vi "BeamAnalyzer.vi"() -> ()   [LabVIEW 2021]
uses:
  <vilib>/vision/Image Controls.llb/IMAQ Image.ctl
  <vilib>/userdefined/High Color/IMAQdx.ctl
  <vilib>/vision/driver/NI_Vision_Acquisition_Software.lvlib
  <vilib>/Utility/TDMS File Viewer/NI_TDMS File Viewer.lvlib
panel:
  in  "tabControl":T1(tab)
  in  "resetOrigin":bool
  in  "setOrigin":bool
  out "lastBufferNumber":u32
  out "imageRows":i32 caption="Rows"
  out "imageCols":i32 caption="Columns"
  out "Trials":i32
  in  "verticalTermPars":cluster{"max iteration":dbl, "tolerance":dbl}={"max iteration"=20.0, "tolerance"=0.0001} caption="Termination \nParameters"
  out "exposureTimeStatus":bool caption="Status"
  in  "aboutButton":bool
  out "vetFitLED":bool
  out "horzFitLED":bool
  in  "maxTrialNumber":i32=10 caption="Max Trial Number"
  out "followCyLED":bool
  out "followCxLED":bool
  in  "exposureTime":dbl caption="Exposure Time" format="%#_6ps"
  out "minMax":u16[](array[numeric]) caption="Min Max Intensities"
  in  "intesityRangeTreshold":dbl=0.33 caption="Intesity Range\nTreshold Fraction"
  in  "fitCol":i32=640
  in  "followCy":bool
  in  "followCx":bool
  in  "stop":bool
  in  "blahButton":bool
  in  "percentageMaxIntensity":dbl=75.0 caption="Percentage Max Intensity" format="%#_g%%"
  out "imageViewer":T2(plugin-control)
  in  "setExposureButton":bool
  in  "horizontalFitButton":bool
  out "horizontal FitPlot":cluster{"xAxis":dbl[], "horizontalFitY":dbl[]}[](graph)
  in  "horizontalTermPars":cluster{"max iteration":dbl, "tolerance":dbl}={"max iteration"=20.0, "tolerance"=0.0001} caption="Termination \nParameters"
  out "horizontalBestFitPars":dbl[](array[numeric]) caption="Best Fit Pars" format="%#_6p"
  out "horizontalFitCovariance":dbl[][](array[numeric]) caption="Covariance" format="%#_6p"
  out "verticalFitPlot":T3(graph)
  out "verticalBestFitPars":dbl[](array[numeric]) caption="Best Fit Pars" format="%#_6p"
  in  "verticalFitButton":bool
  in  "fitRow":i32=480
  out "verticalFitError":errorcluster
  out "horizontalFitError":errorcluster
  in  "saveCurrentImage":bool
  in  "baseName":string="blah"
  in  "basePath":path=path "./"
  out "last Image filename":string
  out "verticalFitCovariance":dbl[][](array[numeric]) caption="Covariance" format="%#_6p"
  out "Cx":dbl caption="X" format="%#_6pm"
  out "Cy":dbl caption="Y" format="%#_6pm"
  out "Y":dbl format="%#_4pm"
  out "X":dbl format="%#_4pm"
  out "centroidCoords":cluster{"Cx":dbl, "Cy":dbl} caption="Centroid Coords" {"Cy" format="%u px"; "Cx" format="%u px"}
  out "wx":dbl format="%#_4pm"
  out "wy":dbl format="%#_4pm"
  out "lumberingLED":bool
  in  "runChartButton":bool
  out "last log filename":string
  in  "log basePath":path
  in  "logBaseName":string="blah"
  in  "logDataButton":bool
  out "wx_wyPlot":cluster{"Numeric":dbl, "Numeric":dbl}(graph)={"Numeric"=24.443322449703377, "Numeric"=50.238781903198756}
  out "CyPlot":dbl(graph)=-0.6586166381835937
  out "CxPlot":dbl(graph)=-1.7079547119140623
  in  "AlliedVisionImageGrabPatch":bool=TRUE
  out "cameraSession":T4 caption="Session Out"
  out "imageBuffer":T2
  in  "reticleColor":u32(colorbox)=3800611 caption="Reticle Pattern Color"
  in  "units":enum32{"um", "mm", "cm"}(radio)
  in  "maxExposureTime":dbl=0.1 caption="Max Exp. Time" format="%#_4ps"
  in  "minExposureTime":dbl=6e-06 caption="Min Exp. Time" format="%#_4ps"
  out "intensityRangeMax":u16
  out "errorExposureTime":errorcluster
  out "errorCameraConfig":errorcluster
  out "errorImageGrab":errorcluster
  out "plotUnitsPrefix":dbl=1000.0
  in  "exposuretimeUnitsPrefix":dbl=1000000.0 caption="Exp.  Time Units Prefix" format="%#_6p"
  out "vendorNameModelName":string
  out "errorCameraParsRequest":errorcluster
  out "IPAddress":string
  in  "nbits":u16=14 min=4 max=15
  in  "pixelSize":dbl=3e-05 caption="Calibrated Pixel Size" format="%#_6pm"
  in  "device":string(combo)="cam1"
  out "xAxis":dbl[](array[numeric])
  out "yAxis":dbl[](array[numeric])
  out "colsOffset":i32
  out "rowsOffset":i32
  out "rowArray":u16[](array[numeric])
  out "colArray":u16[](array[numeric])
  out "verticalFitY":dbl[](array[numeric])
  out "horizontalFitY":dbl[](array[numeric])
  out "centroidError":errorcluster
  out "imageDecorated":T2
  out "TDMS_Location":path
  out "TDMS_Handle":refnum<k34>
  out "errorTDMS_LogClose":errorcluster
  out "errorTDMS_LogOpen":errorcluster
  out "yAxisScaled":dbl[](array[numeric])
  out "xAxisScaled":dbl[](array[numeric])
  out "errorTDMS_LogWrite":errorcluster
  # "I0"
  # "AU/px"
  # "m"
  # "x0"
  # "m"
  # "w0"
  # "AU/px"
  # "I1"
  # "Exposure Setting"
  # "Centroid"
  # "Image Statistics"
  # "Save Current Livefeed Image"
  # "AU/px"
  # "I0"
  # "m"
  # "x0"
  # "w0"
  # "m"
  # "AU/px"
  # "I1"
  # "Spot Radii"
  # "Centroid Coords"
  # "Camera Configuration"
  # "Model"
  # "Plot Configuration"
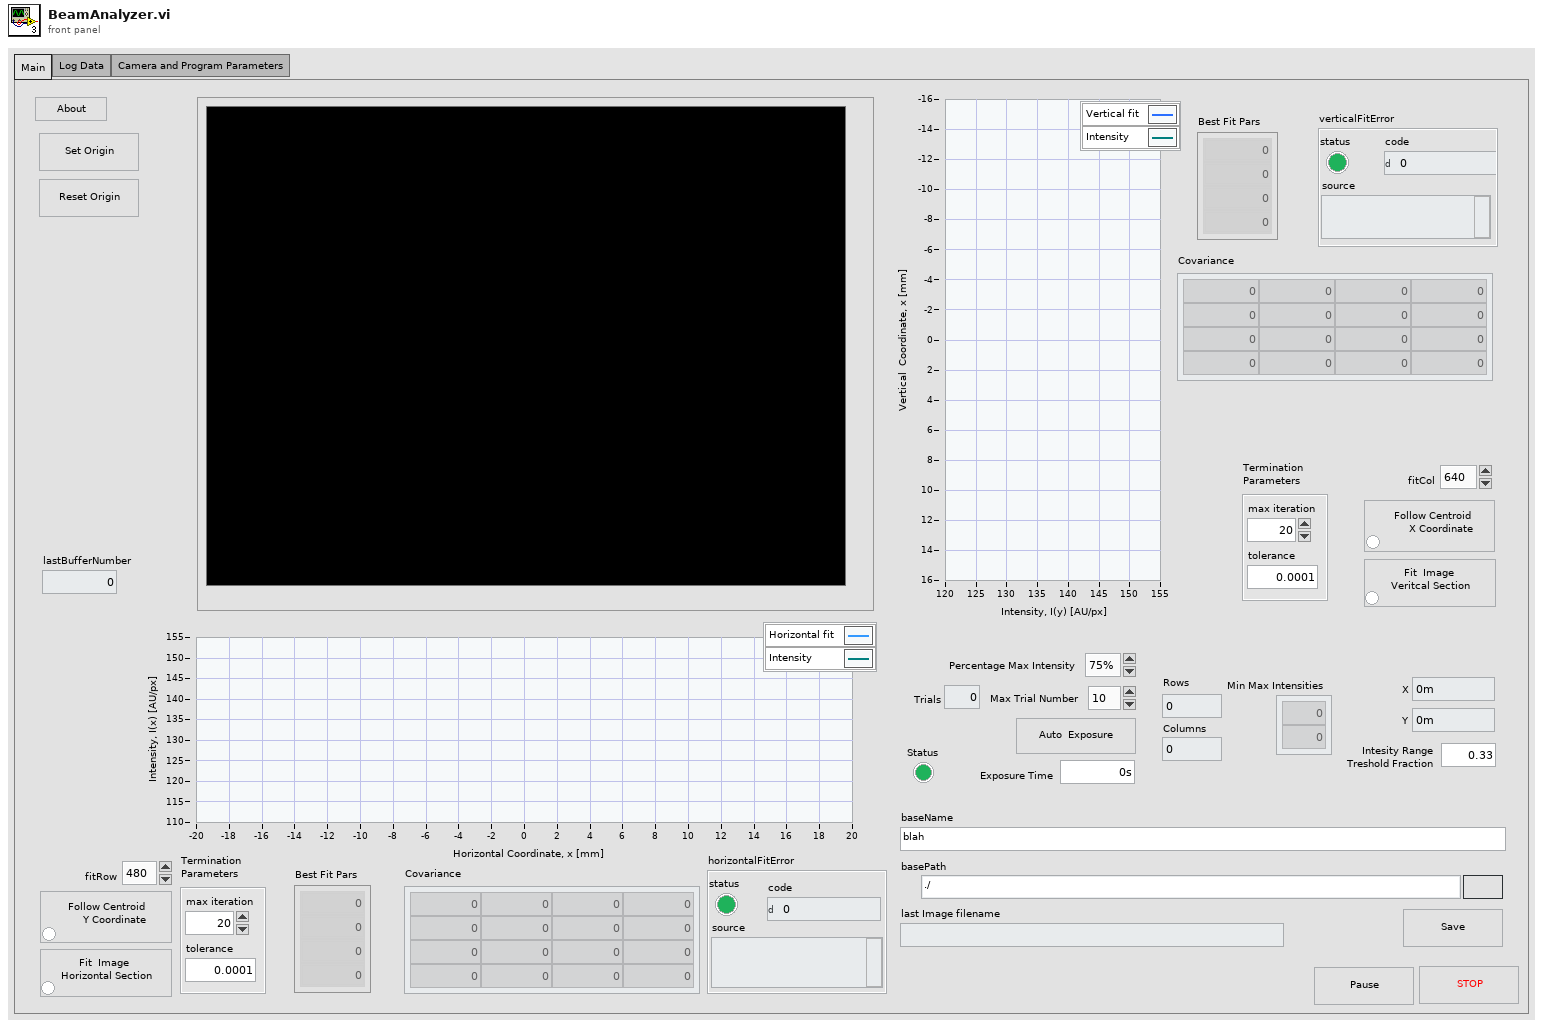
[diagram p1: front panel]
types:
  T1 = enum32{"Main", "Log Data", "Camera and Program Parameters"}
  T2 = typedef "IMAQ Image.ctl" = refnum<image>
  T3 = cluster{"best nonlinear fit":dbl[], "yAxis":dbl[]}[]
  T4 = typedef "IMAQdx.ctl" = refnum<k21>
  T5 = enum32{"Fit", "Log Data", "Camera and Program Parameters"}
  T6 = enum32{"Fit", "Log Data", "Hardware  Parameters"}
  T7 = enum16{"open", "open or create", "create or replace", "create", "open (read-only)"}
  T8 = cluster{"xAxisScaled":dbl[], "horizontalFitY":dbl[]}
  T9 = cluster{"xAxisScaled":dbl[], "horizontalFitY":dbl[]}[]
  T10 = cluster{"verticalFitY":dbl[], "yAxisScaled":dbl[]}
  T11 = cluster{"verticalFitY":dbl[], "yAxisScaled":dbl[]}[]
  T12 = typedef "NI_Matrix.lvlib/RealMatrix.ctl" = dbl[][]
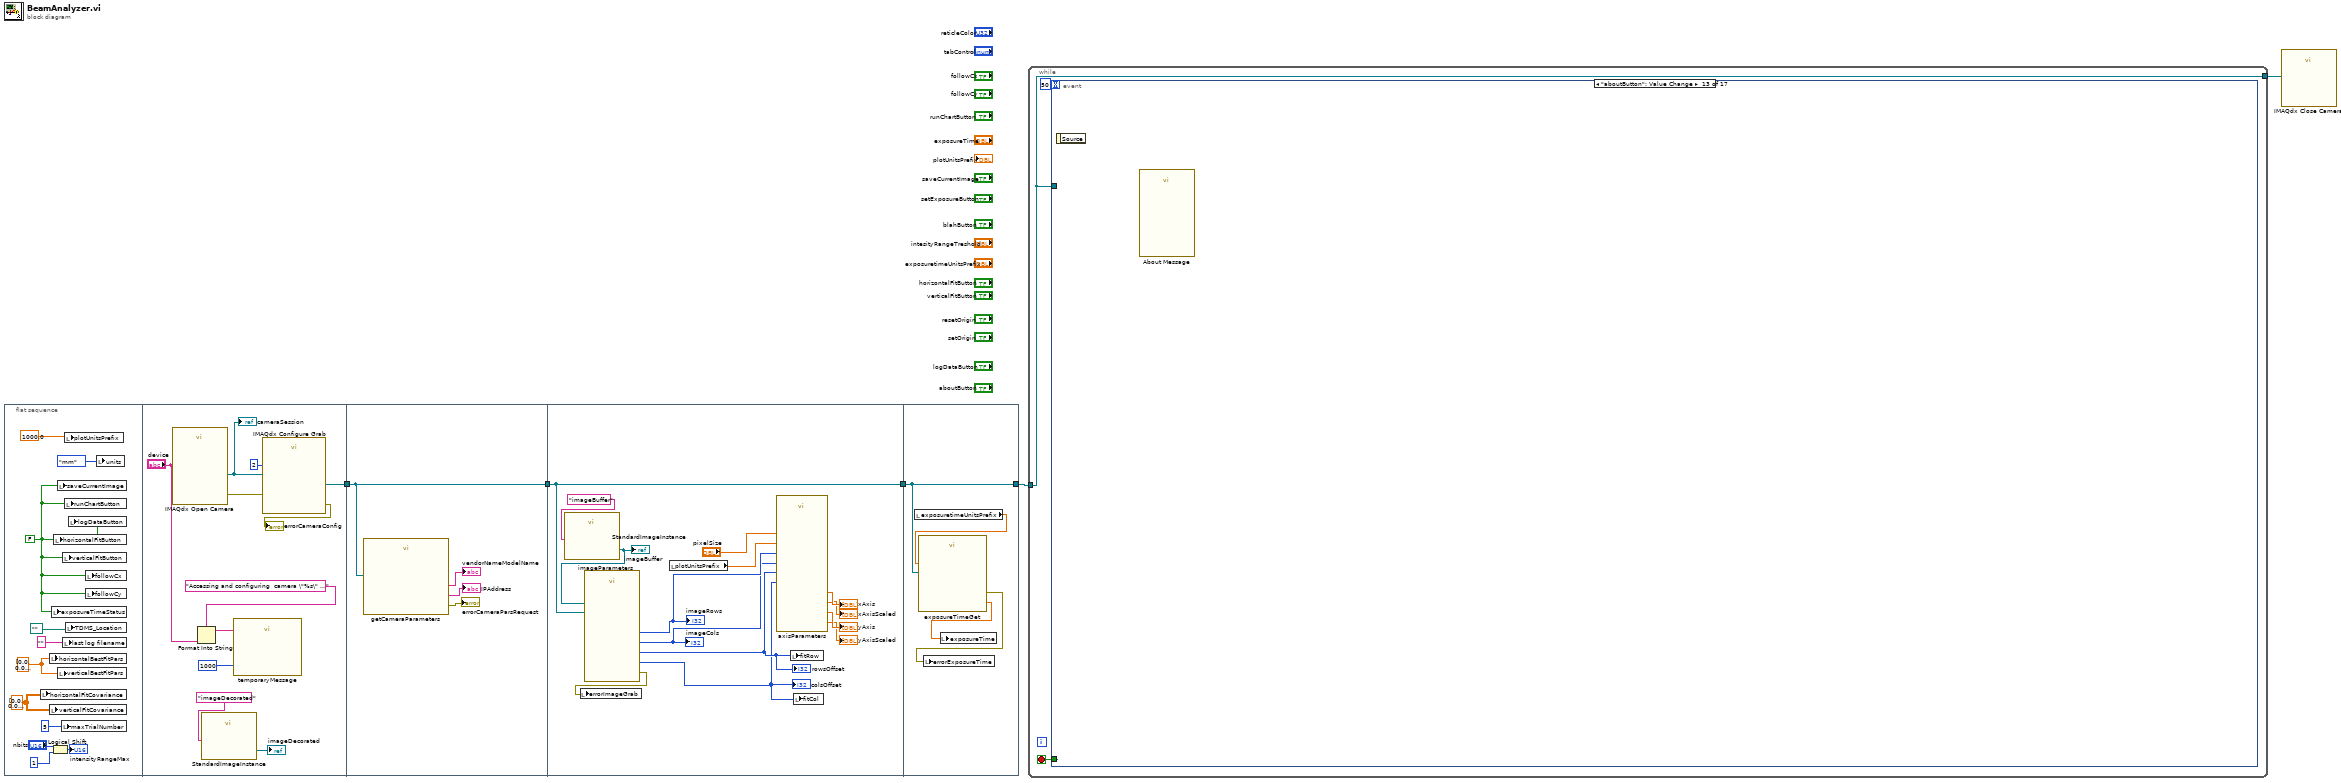
[diagram p0: block diagram]
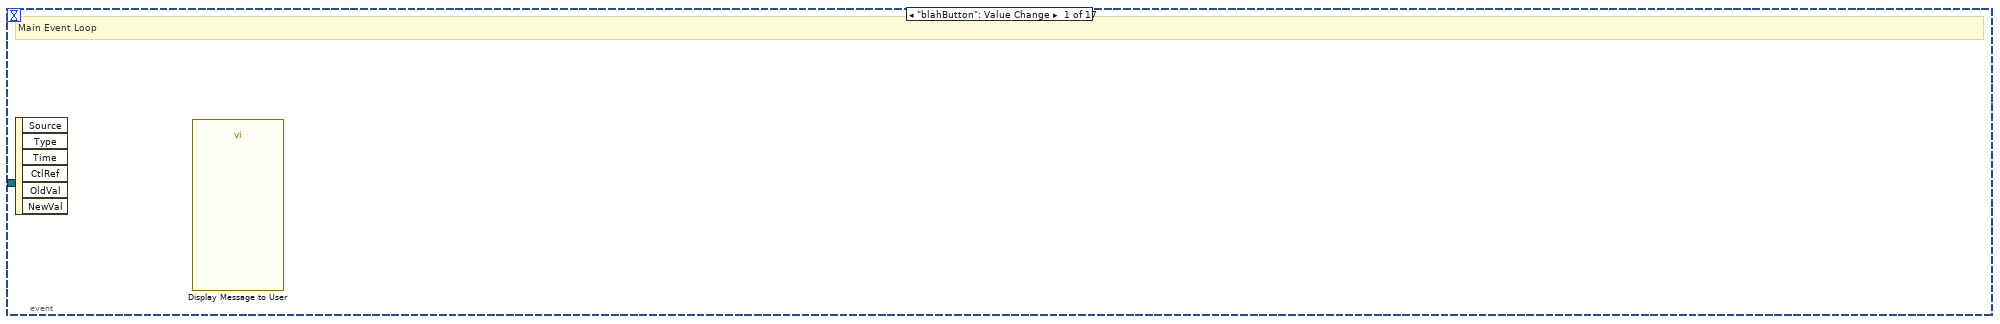
[diagram p2: hidden frame]
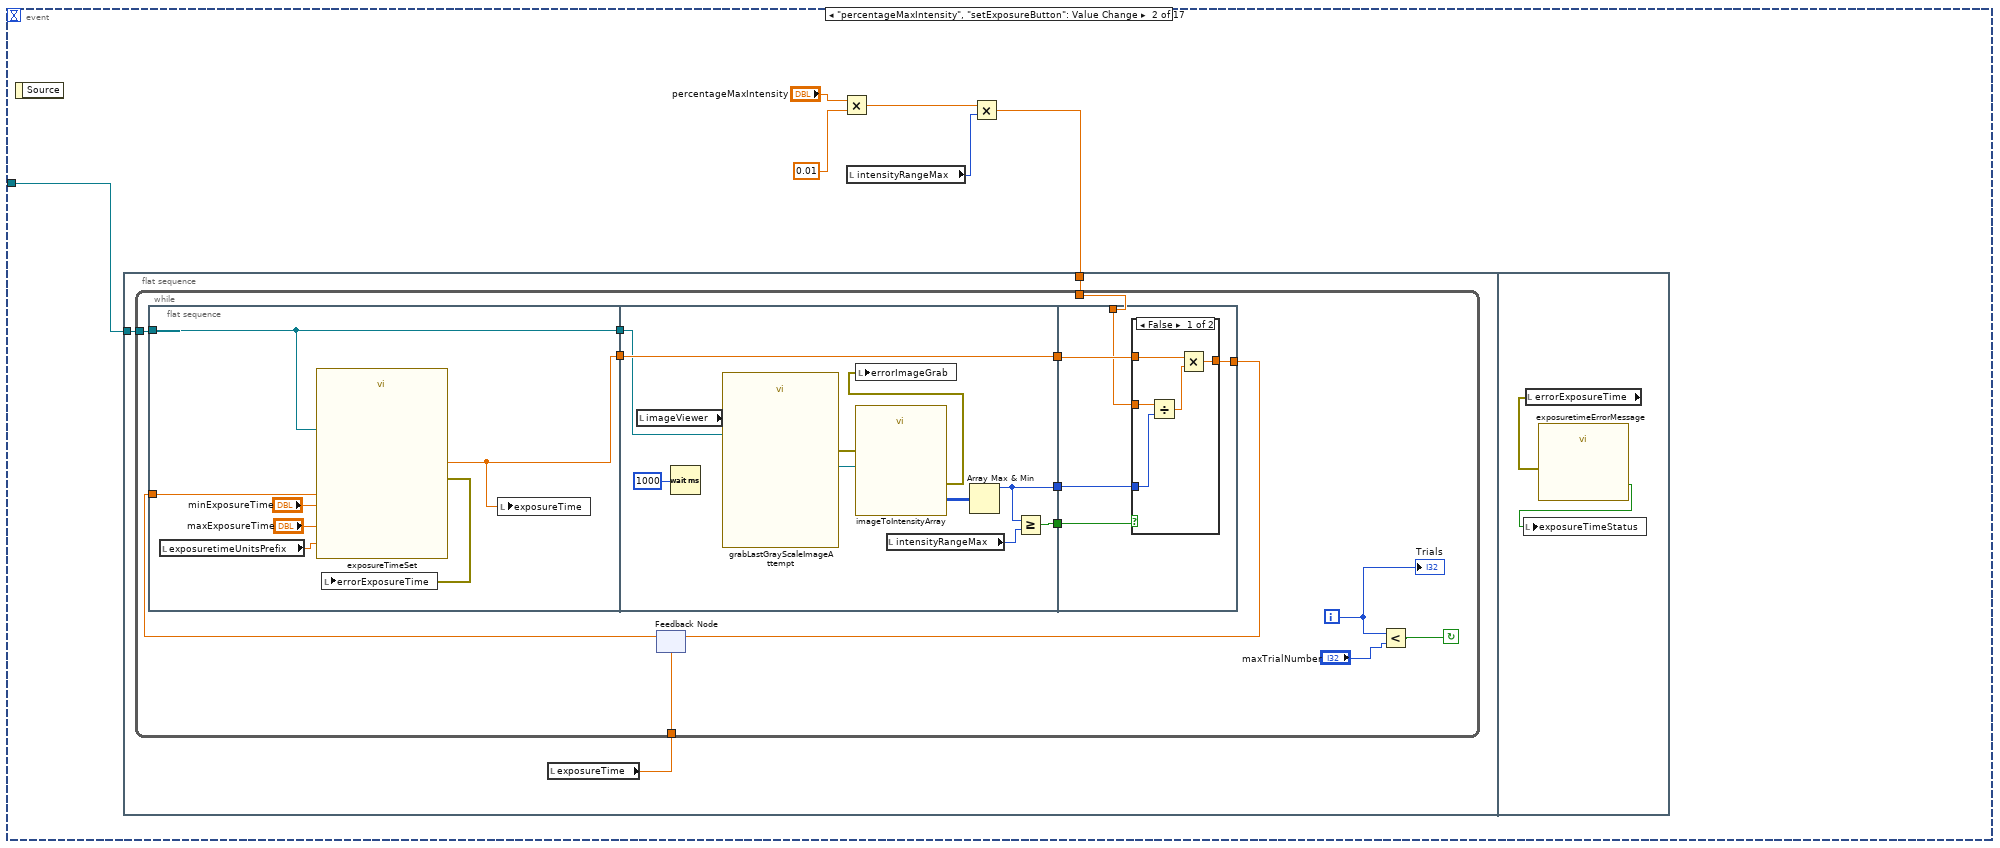
[diagram p3: hidden frame]
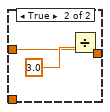
[diagram p4: hidden frame]
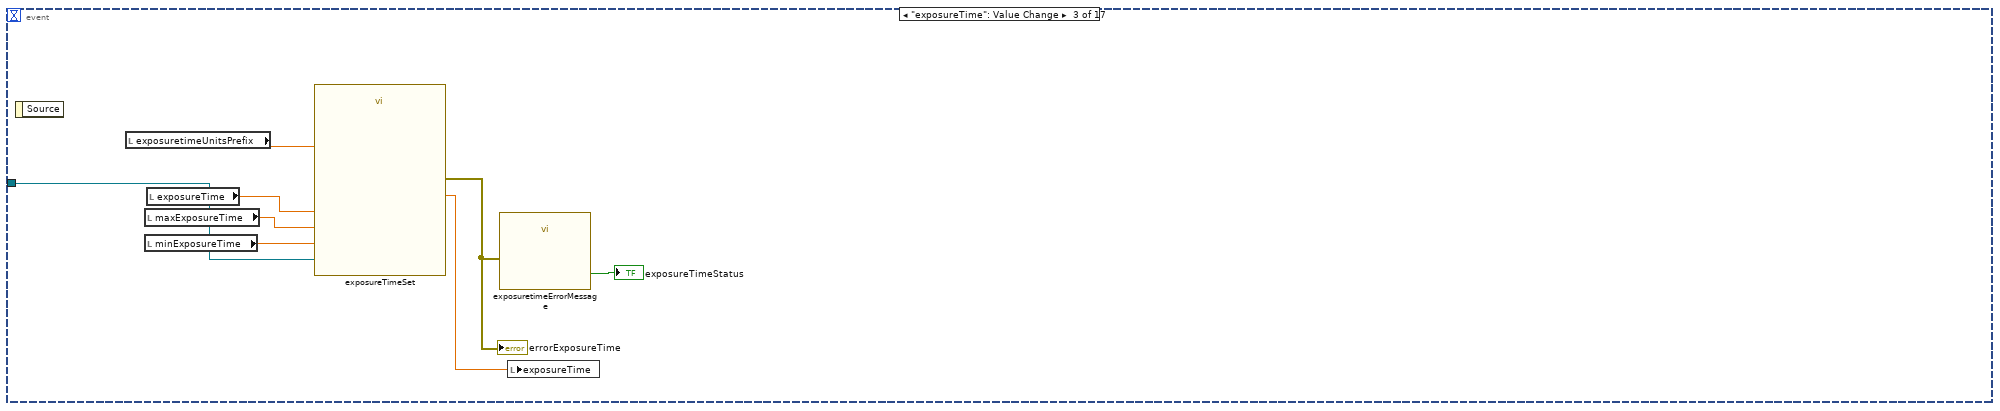
[diagram p5: hidden frame]
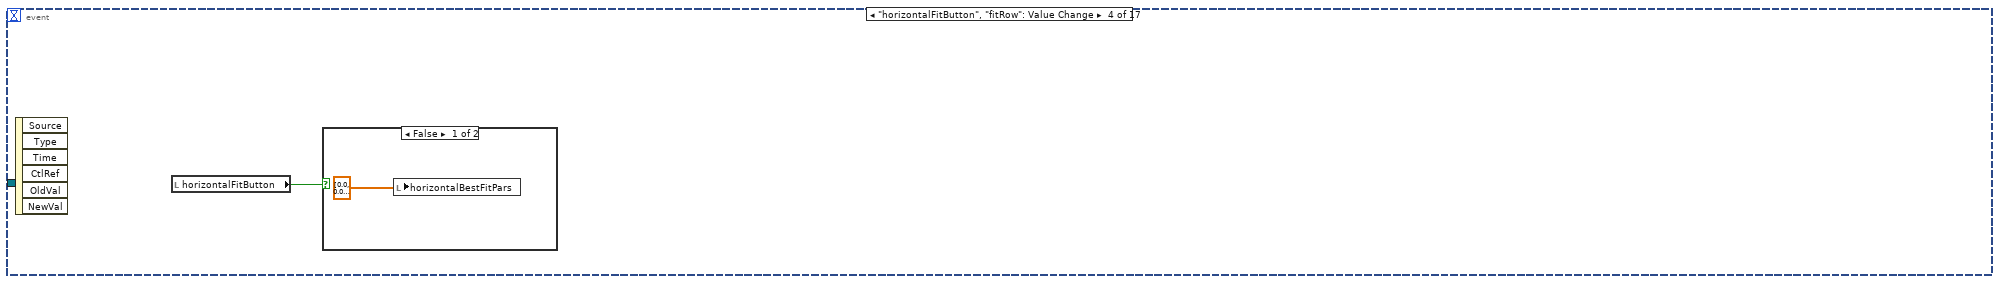
[diagram p6: hidden frame]
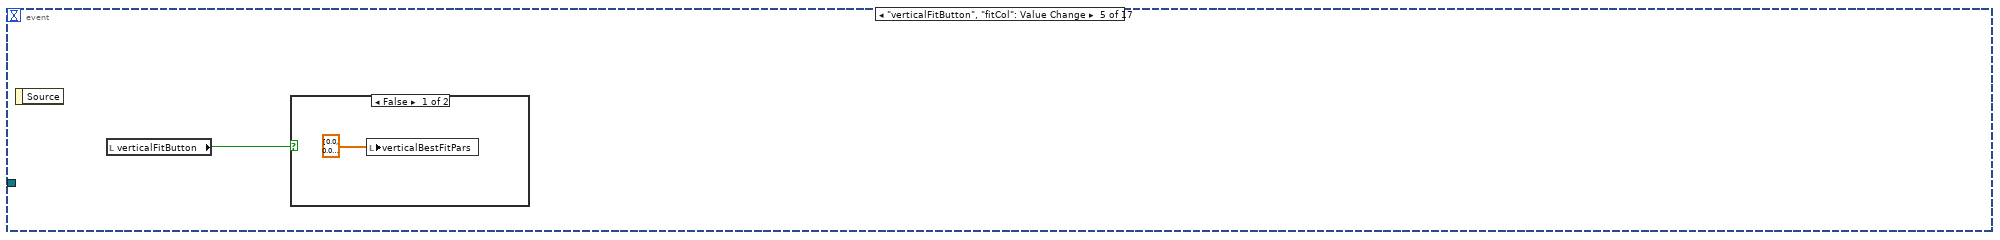
[diagram p8: hidden frame]
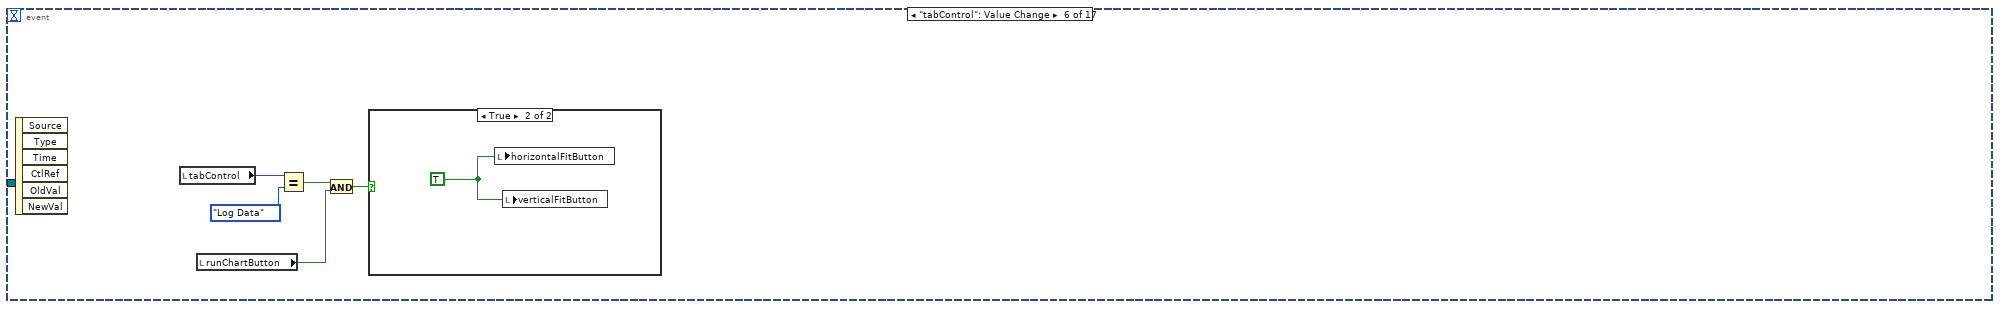
[diagram p10: hidden frame]
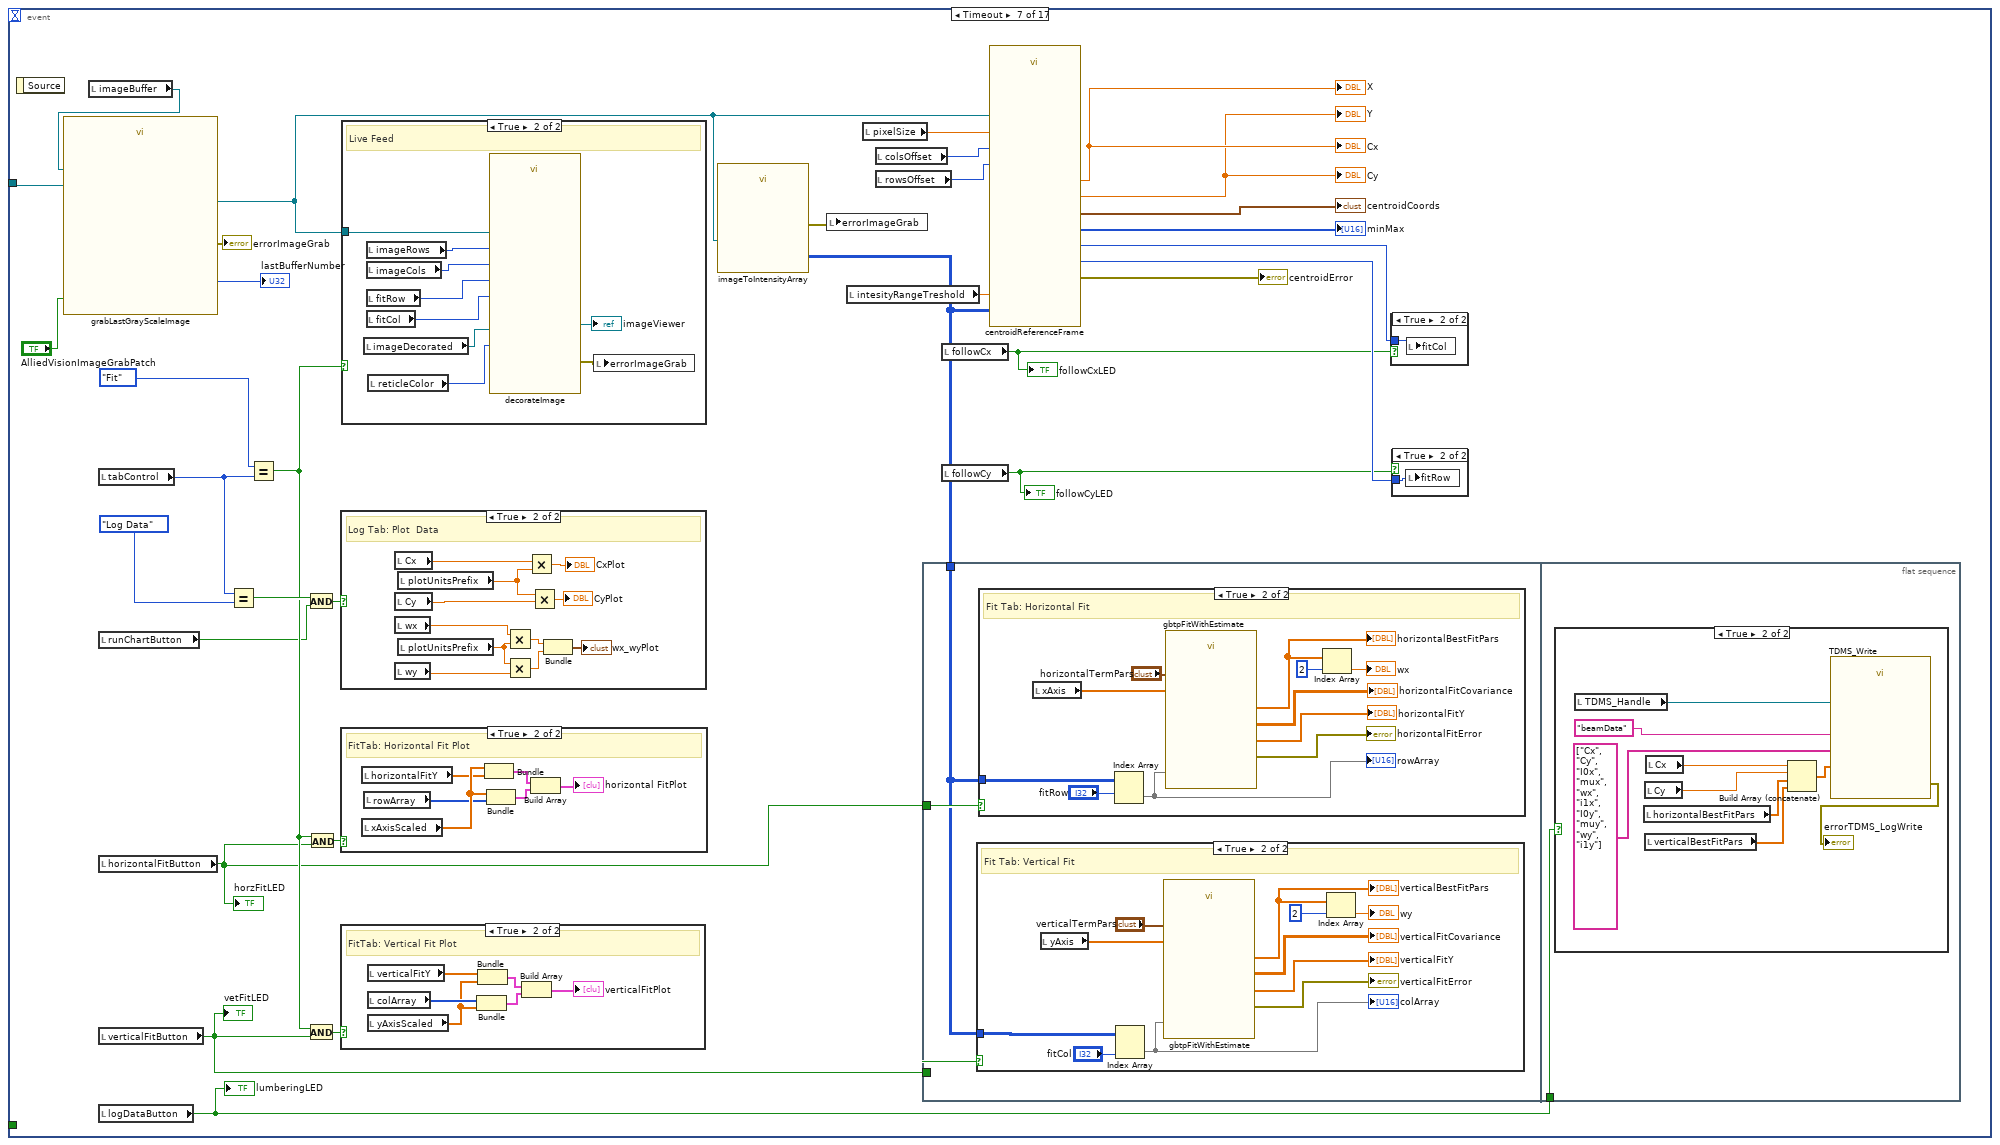
[diagram p12: hidden frame]
diagram:
  n1 = flat-sequence {
    tunnel: [w23] -> w3
    tunnel: [w28] -> w4
    tunnel: w3 -> [w28]
    tunnel: [w42] -> w5
    tunnel: w4 -> [w42]
    tunnel: [w46] -> w2
    tunnel: w5 -> [w46]
    frame #0 {
      w13 = dbl[][] [[0.0, 0.0, 0.0, 0.0], [0.0, 0.0, 0.0, 0.0], [0.0, 0.0, 0.0, 0.0], [0.0, 0.0, 0.0, 0.0]] ("horizontalFitCovariance")
      w14 = dbl[] [0.0, 0.0, 0.0, 0.0, 0.0] ("horizontalBestFitPars")
      w11 = FALSE
      n2 = local write "horizontalFitCovariance"(w13) -> ()
      n3 = local write "horizontalBestFitPars"(w14) -> ()
      n4 = local write "verticalFitCovariance"(w13) -> ()
      n5 = local write "exposureTimeStatus"(w11) -> ()
      n6 = Logical Shift(y="nbits", x=i16 1 ("y")) -> (x << y=→"intensityRangeMax":i16)
      n7 = local write "horizontalFitButton"(w11) -> ()
      n8 = local write "saveCurrentImage"(w11) -> ()
      n9 = local write "verticalBestFitPars"(w14) -> ()
      n10 = local write "maxTrialNumber"(5 ("maxTrialNumber")) -> ()
      n11 = local write "verticalFitButton"(w11) -> ()
      n12 = local write "last log filename"("" ("last Image filename")) -> ()
      n13 = local write "plotUnitsPrefix"(1000.0) -> ()
      n14 = local write "runChartButton"(w11) -> ()
      n15 = local write "TDMS_Location"(path "" ("TDMS_Location")) -> ()
      n16 = local write "logDataButton"(w11) -> ()
      n17 = local write "followCx"(w11) -> ()
      n18 = local write "followCy"(w11) -> ()
      n19 = local write "units"(enum32{"um", "mm", "cm"}."mm" ("units")) -> ()
    }
    frame #1 {
      n20 = call <vilib>:"IMAQdx Open Camera.vi"("Session In"="device") -> ("error out"=w27:errorcluster, "Session Out"=w24:T4)  [unwired: 9 in]
      "cameraSession" <- w24
      n21 = Format Into String(format string="Accessing and configuring  camera \"%s\" ..." ("string"), "device") -> (resulting string=w22:string)  [unwired: 2 in, 1 out]
      n22 = call "StandardImageInstance.vi"("Image Name"="imageDecorated") -> ("Refnum out"=→"imageDecorated":T2)  [unwired: 10 in]
      n23 = call "temporaryMessage.vi"("milliseconds to wait"=u32 1000, "message"=w22) -> ()  [unwired: 1 in]
      n24 = call <vilib>:"IMAQdx Configure Grab.vi"("error in"=w27, "Number of Buffers"=u32 2, "Session In"=w24) -> ("error out"=→"errorCameraConfig":errorcluster, "Session Out"=w23:T4)  [unwired: 7 in]
    }
    frame #2 {
      n25 = call "getCameraParameters.vi"("IMAQdx Session"=w28) -> ("errorCameraParsRequest"=→"errorCameraParsRequest":errorcluster, "VendorNameModelName"=→"vendorNameModelName":string, "IPAddress"=→"IPAddress":string)  [unwired: 8 in]
    }
    frame #3 {
      n26 = call "StandardImageInstance.vi"("Image Name"="imageBuffer") -> ("Refnum out"=w43:T2)  [unwired: 10 in]
      "imageBuffer" <- w43
      n27 = call "imageParameters.vi"("sessionIn"=w42, "imageIn"=w43) -> ("imageHalfRows"=w33:i32, "imageHalfCols"=w32:i32, "imageCols"=w34:i32, "imageRows"=w35:i32, "errorImageGrab"=w45:errorcluster)  [unwired: 5 in]
      "imageRows" <- w35
      "imageCols" <- w34
      "colsOffset" <- w32
      "rowsOffset" <- w33
      n28 = local write "errorImageGrab"(w45) -> ()
      n29 = local read "plotUnitsPrefix"() -> (w36:dbl)
      n30 = call "axisParameters.vi"("colOffset"=w32, "rowOffset"=w33, "cols"=w34, "rows"=w35, "pixelSize"="pixelSize", "plotUnitsPrefix"=w36) -> ("yAxisScaled"=→"yAxisScaled":dbl[], "xAxisScaled"=→"xAxisScaled":dbl[], "yAxis"=→"yAxis":dbl[], "xAxis"=→"xAxis":dbl[])
      n31 = local write "fitRow"(w33) -> ()
      n32 = local write "fitCol"(w32) -> ()
    }
    frame #4 {
      n33 = local read "exposuretimeUnitsPrefix"() -> (w47:dbl)
      n34 = call "exposureTimeGet.vi"("exposureUnitsPrefix"=w47, "Session in"=w46) -> ("errorOut"=w49:errorcluster, "exposureTime"=w48:dbl)  [unwired: 2 in]
      n35 = local write "errorExposureTime"(w49) -> ()
      n36 = local write "exposureTime"(w48) -> ()
    }
  }
  n37 = while {
    tunnel: w2 -> [w50]
    tunnel: [w50] -> w1
    stop <- w52 stop-if-true
    n38 = event shown="[12] \"aboutButton\": Value Change" {
      selector: _ -> [_ _ _ _ _ _ _ _ _ _ _ _ _ _ _ _ _]
      dyn-events: _ -> [_ _ _ _ _ _ _ _ _ _ _ _ _ _ _ _ _]
      timeout: 50 -> [_ _ _ _ _ _ _ _ _ _ _ _ _ _ _ _ _]
      tunnel: [_ _ _ _ _ _ _ _ _ _ _ _ _ _ _ _ "stop"] -> w52
      tunnel: w50 -> [_ w53 w108 _ _ _ w130 _ _ _ _ _ _ _ _ _ _]
      event "blahButton": Value Change {
        # "Main Event Loop"
        n39 = event-data() -> ()  [unwired: 1 in, 6 out]
        n40 = call "Display Message to User"() -> ()  [unwired: 10 in, 2 out]
      }
      event "percentageMaxIntensity", "setExposureButton": Value Change {
        n41 = event-data() -> ()  [unwired: 1 in, 1 out]
        n42 = flat-sequence {
          tunnel: w56 -> [w61]
          tunnel: w53 -> [w60]
          frame #0 {
            n43 = local read "exposureTime"() -> (w59:dbl)
            n44 = while {
              tunnel: w61 -> [w74]
              tunnel: w60 -> [w69]
              tunnel: w59 -> [w62]
              i -> [w67]
              stop <- w65 continue-if-true
              n45 = flat-sequence {
                tunnel: [w75] -> w71
                tunnel: w69 -> [w77]
                tunnel: [w77] -> w68
                tunnel: w63 -> [w76]
                tunnel: [w92] -> w73
                tunnel: [w90] -> w72
                tunnel: w71 -> [w92]
                tunnel: [w84] -> w70
                tunnel: w68 -> [w83]
                tunnel: w73 -> [w97]
                tunnel: w74 -> [w96]
                tunnel: [w95] -> w64
                tunnel: w72 -> [w94]
                tunnel: w70 -> [w93]
                frame #0 {
                  n46 = local read "exposuretimeUnitsPrefix"() -> (w81:dbl)
                  n47 = call "exposureTimeSet.vi"("exposureTime (s)"=w76, "maxExposureTime"="minExposureTime", "minExposureTime"="maxExposureTime", "exposureUnitsPrefix"=w81, "sessionIn"=w77) -> ("error out"=w80:errorcluster, "exposureTimeReadback"=w75:dbl)  [unwired: 3 in]
                  n48 = local write "errorExposureTime"(w80) -> ()
                  n49 = local write "exposureTime"(w75) -> ()
                }
                frame #1 {
                  n50 = local read "imageViewer"() -> (w85:T2)
                  n51 = Wait (ms)(milliseconds to wait=u32 1000) -> ()  [unwired: 1 out]
                  n52 = call "grabLastGrayScaleImageAttempt.vi"("ImageInstance"=w85, "SessionIn"=w83) -> ("ImageOut"=w89:T2, "errorOut"=w88:errorcluster)  [unwired: 2 in, 2 out]
                  n53 = call "imageToIntensityArray.vi"("errorIn"=w88, "image"=w89) -> ("erorOut"=w87:errorcluster, "imageArray"=w86:u16[][])
                  n54 = local write "errorImageGrab"(w87) -> ()
                  n55 = local read "intensityRangeMax"() -> (w91:u16)
                  n56 = Array Max & Min(array=w86) -> (max value=w84:u16)  [unwired: 3 out]
                  n57 = Greater Or Equal?(x=w84, y=w91) -> (x >= y?=w90:bool)
                }
                frame #2 {
                  n58 = case shown="False" w94 {
                    tunnel: w96 -> [w101 _]
                    tunnel: [w98 w104] -> w95
                    tunnel: w97 -> [w99 w103]
                    tunnel: w93 -> [w102 _]
                    frame False {
                      n59 = Divide(x=w101, y=w102) -> (x/y=w100:dbl)
                      n60 = Multiply(x=w99, y=w100) -> (x*y=w98:dbl)
                    }
                    frame True {
                      n61 = Divide(x=w103, y=3.0) -> (x/y=w104:dbl)
                    }
                  }
                }
              }
              n62 = feedback-in #1(w64) -> ()
              n63 = feedback #1(w62) -> (w63:dbl)
              n64 = Less?(x=w67, y="maxTrialNumber") -> (x < y?=w65:bool)
              "Trials" <- w67
            }
          }
          frame #1 {
            n65 = local read "errorExposureTime"() -> (w107:errorcluster)
            n66 = call "exposuretimeErrorMessage.vi"("errorIn"=w107) -> ("exposureTimeStatus"=w106:bool)  [unwired: 10 in]
            n67 = local write "exposureTimeStatus"(w106) -> ()
          }
        }
        n68 = Multiply(x="percentageMaxIntensity", y=0.01) -> (x*y=w55:dbl)
        n69 = local read "intensityRangeMax"() -> (w54:u16)
        n70 = Multiply(x=w55, y=w54) -> (x*y=w56:dbl)
      }
      event "exposureTime": Value Change {
        n71 = event-data() -> ()  [unwired: 1 in, 1 out]
        n72 = local read "exposuretimeUnitsPrefix"() -> (w109:dbl)
        n73 = local read "maxExposureTime"() -> (w111:dbl)
        n74 = local read "minExposureTime"() -> (w110:dbl)
        n75 = local read "exposureTime"() -> (w112:dbl)
        n76 = call "exposureTimeSet.vi"("exposureTime (s)"=w112, "maxExposureTime"=w111, "minExposureTime"=w110, "exposureUnitsPrefix"=w109, "sessionIn"=w108) -> ("error out"=w114:errorcluster, "exposureTimeReadback"=w115:dbl)  [unwired: 3 in]
        "errorExposureTime" <- w114
        n77 = call "exposuretimeErrorMessage.vi"("errorIn"=w114) -> ("exposureTimeStatus"=→"exposureTimeStatus":bool)  [unwired: 10 in]
        n78 = local write "exposureTime"(w115) -> ()
      }
      event "horizontalFitButton", "fitRow": Value Change {
        n79 = event-data() -> ()  [unwired: 1 in, 6 out]
        n80 = local read "horizontalFitButton"() -> (w116:bool)
        n81 = case shown="False" w116 {
          frame False {
            n82 = local write "horizontalBestFitPars"(dbl[] [0.0, 0.0, 0.0, 0.0, 0.0] ("horizontalBestFitPars")) -> ()
          }
          frame True {
          }
        }
      }
      event "verticalFitButton", "fitCol": Value Change {
        n83 = event-data() -> ()  [unwired: 1 in, 1 out]
        n84 = local read "verticalFitButton"() -> (w118:bool)
        n85 = case shown="False" w118 {
          frame False {
            n86 = local write "verticalBestFitPars"(dbl[] [0.0, 0.0, 0.0, 0.0, 0.0] ("horizontalBestFitPars")) -> ()
          }
          frame True {
          }
        }
      }
      event "tabControl": Value Change {
        n87 = event-data() -> ()  [unwired: 1 in, 6 out]
        n88 = local read "tabControl"() -> (w120:T1)
        n89 = local read "runChartButton"() -> (w121:bool)
        n90 = Equal?(x=w120, y=T5."Log Data") -> (x = y?=w122:bool)
        n91 = And(x=w122, y=w121) -> (x .and. y?=w123:bool)
        n92 = case shown="True" w123 {
          frame False {
          }
          frame True {
            w125 = TRUE
            n93 = local write "horizontalFitButton"(w125) -> ()
            n94 = local write "verticalFitButton"(w125) -> ()
          }
        }
      }
      event Timeout {
        n95 = event-data() -> ()  [unwired: 1 in, 1 out]
        n96 = local read "imageBuffer"() -> (w129:T2)
        n97 = call "grabLastGrayScaleImage.vi"("ImageInstance"=w129, "AlliedVisionImageGrabPatch"="AlliedVisionImageGrabPatch", "SessionIn"=w130) -> ("ImageOut"=w136:T2, "errorOut"=→"errorImageGrab":errorcluster, "bufferNumberActual"=→"lastBufferNumber":u32)  [unwired: 2 in, 1 out]
        n98 = local read "tabControl"() -> (w138:T1)
        n99 = local read "runChartButton"() -> (w139:bool)
        n100 = local read "horizontalFitButton"() -> (w134:bool)
        "horzFitLED" <- w134
        n101 = local read "verticalFitButton"() -> (w133:bool)
        "vetFitLED" <- w133
        n102 = local read "logDataButton"() -> (w137:bool)
        "lumberingLED" <- w137
        n103 = Equal?(x=w138, y=T6."Log Data") -> (x = y?=w152:bool)
        n104 = Equal?(x=T6."Fit" ("y"), y=w138) -> (x = y?=w149:bool)
        n105 = And(x=w152, y=w139) -> (x .and. y?=w157:bool)
        n106 = And(x=w149, y=w133) -> (x .and. y?=w145:bool)
        n107 = And(x=w149, y=w134) -> (x .and. y?=w150:bool)
        n108 = case shown="True" w157 {
          frame False {
          }
          frame True {
            # "Log Tab: Plot  Data"
            n109 = local read "Cx"() -> (w223:dbl)
            n110 = local read "Cy"() -> (w222:dbl)
            n111 = local read "wx"() -> (w218:dbl)
            n112 = local read "wy"() -> (w217:dbl)
            n113 = local read "plotUnitsPrefix"() -> (w225:dbl)
            n114 = local read "plotUnitsPrefix"() -> (w219:dbl)
            n115 = Multiply(x=w218, y=w219) -> (x*y=w221:dbl)
            n116 = Multiply(x=w219, y=w217) -> (x*y=w220:dbl)
            n117 = Multiply(x=w223, y=w225) -> (x*y=→"CxPlot":dbl)
            n118 = Multiply(x=w225, y=w222) -> (x*y=→"CyPlot":dbl)
            n119 = Bundle(w221, w220) -> (→"wx_wyPlot":cluster{dbl, dbl})  [unwired: 1 in]
          }
        }
        n120 = case shown="True" w150 {
          frame False {
          }
          frame True {
            # "FitTab: Horizontal Fit Plot"
            n121 = local read "horizontalFitY"() -> (w204:dbl[])
            n122 = local read "xAxisScaled"() -> (w205:dbl[])
            n123 = local read "rowArray"() -> (w203:u16[])
            n124 = Bundle("xAxisScaled"=w205, "horizontalFitY"=w204) -> (w207:T8)  [unwired: 1 in]
            n125 = Bundle("xAxisScaled"=w205, "rowArray"=w203) -> (w206:cluster{"xAxisScaled":dbl[], "rowArray":u16[]})  [unwired: 1 in]
            n126 = Build Array(w207, w206) -> (→"horizontal FitPlot":T9)
          }
        }
        n127 = case shown="True" w145 {
          frame False {
          }
          frame True {
            # "FitTab: Vertical Fit Plot"
            n128 = local read "verticalFitY"() -> (w197:dbl[])
            n129 = local read "colArray"() -> (w199:u16[])
            n130 = local read "yAxisScaled"() -> (w196:dbl[])
            n131 = Bundle("colArray"=w199, "yAxisScaled"=w196) -> (w198:cluster{"colArray":u16[], "yAxisScaled":dbl[]})  [unwired: 1 in]
            n132 = Bundle("verticalFitY"=w197, "yAxisScaled"=w196) -> (w195:T10)  [unwired: 1 in]
            n133 = Build Array(w195, w198) -> (→"verticalFitPlot":T11)
          }
        }
        n134 = case shown="True" w149 {
          tunnel: w136 -> [_ w213]
          frame False {
          }
          frame True {
            # "Live Feed"
            n135 = local read "imageDecorated"() -> (w209:T2)
            n136 = local read "imageRows"() -> (w212:i32)
            n137 = local read "imageCols"() -> (w211:i32)
            n138 = local read "fitRow"() -> (w214:i32)
            n139 = local read "fitCol"() -> (w215:i32)
            n140 = local read "reticleColor"() -> (w208:u32)
            n141 = call "decorateImage.vi"("reticleColor"=w208, "imageRows"=w212, "FitCol"=w215, "ImageDest"=w209, "FitRow"=w214, "imageCols"=w211, "image"=w213) -> ("error out"=w210:errorcluster, "imageDecorated"=→"imageViewer":T2)  [unwired: 3 in]
            n142 = local write "errorImageGrab"(w210) -> ()
          }
        }
        n143 = call "imageToIntensityArray.vi"("image"=w136) -> ("erorOut"=w128:errorcluster, "imageArray"=w135:u16[][])  [unwired: 1 in]
        n144 = local write "errorImageGrab"(w128) -> ()
        n145 = local read "intesityRangeTreshold"() -> (w142:dbl)
        n146 = local read "pixelSize"() -> (w154:dbl)
        n147 = local read "colsOffset"() -> (w156:i32)
        n148 = local read "rowsOffset"() -> (w155:i32)
        n149 = flat-sequence {
          tunnel: w134 -> [w161]
          tunnel: w133 -> [w160]
          tunnel: w135 -> [w159]
          tunnel: w137 -> [w184]
          frame #0 {
            n150 = case shown="True" w160 {
              tunnel: w159 -> [_ w176]
              frame False {
              }
              frame True {
                # "Fit Tab: Vertical Fit"
                n151 = local read "yAxis"() -> (w182:dbl[])
                n152 = Index Array(array=w176, index (col)="fitCol") -> (element=w174:u16[])  [unwired: 1 in]
                "colArray" <- w174
                n153 = call "gbtpFitWithEstimate.vi"("X"=w182, "terminationPars"="verticalTermPars", "imageArray"=w174) -> ("errorOut"=→"verticalFitError":errorcluster, "fitPars"=w180:dbl[], "fitCovariance"=→"verticalFitCovariance":T12, "fitY"=→"verticalFitY":dbl[])  [unwired: 2 in]
                "verticalBestFitPars" <- w180
                n154 = Index Array(array=w180, index=2) -> (element=→"wy":dbl)
              }
            }
            n155 = case shown="True" w161 {
              tunnel: w159 -> [_ w170]
              frame False {
              }
              frame True {
                # "Fit Tab: Horizontal Fit"
                n156 = local read "xAxis"() -> (w166:dbl[])
                n157 = Index Array(array=w170, index (row)="fitRow") -> (element=w168:u16[])  [unwired: 1 in]
                "rowArray" <- w168
                n158 = call "gbtpFitWithEstimate.vi"("X"=w166, "terminationPars"="horizontalTermPars", "imageArray"=w168) -> ("errorOut"=→"horizontalFitError":errorcluster, "fitPars"=w165:dbl[], "fitCovariance"=→"horizontalFitCovariance":T12, "fitY"=→"horizontalFitY":dbl[])  [unwired: 2 in]
                "horizontalBestFitPars" <- w165
                n159 = Index Array(array=w165, index=2) -> (element=→"wx":dbl)
              }
            }
          }
          frame #1 {
            n160 = case shown="True" w184 {
              frame False {
              }
              frame True {
                n161 = local read "TDMS_Handle"() -> (w192:refnum<k34>)
                n162 = local read "horizontalBestFitPars"() -> (w186:dbl[])
                n163 = local read "Cy"() -> (w189:dbl)
                n164 = local read "verticalBestFitPars"() -> (w185:dbl[])
                n165 = local read "Cx"() -> (w193:dbl)
                n166 = Build Array (concatenate)(w193, w189, w186, w185) -> (w188:dbl[])
                n167 = call "TDMS_Write.vi"("namesArray"=string[] ["Cx", "Cy", "I0x", "mux", "wx", "i1x", "I0y", "muy", "wy", "i1y"], "Array - Numeric"=w188, "groupName"="beamData" ("group name in (Untitled)"), "TDMS_HandleIn"=w192) -> ("errorTDMS_Write"=→"errorTDMS_LogWrite":errorcluster)  [unwired: 1 out]
              }
            }
          }
        }
        n168 = local read "followCx"() -> (w141:bool)
        "followCxLED" <- w141
        n169 = local read "followCy"() -> (w140:bool)
        "followCyLED" <- w140
        n170 = call "centroidReferenceFrame.vi"("yOffset"=w155, "image"=w136, "imageArray"=w135, "xOffset"=w156, "percentOffset"=w142, "exffectivePiixelSize"=w154) -> ("errorOut"=→"centroidError":errorcluster, "row"=w147:u16, "Cx"=→"Cx" →"X":dbl, "Cy"=→"Cy" →"Y":dbl, "centroid"=→"centroidCoords":cluster{"X Centroid":sgl, "Y Centroid":sgl}, "col"=w146:u16, "minMax"=→"minMax":u16[])  [unwired: 3 in]
        n171 = case shown="True" w141 {
          tunnel: w146 -> [_ w201]
          frame False {
          }
          frame True {
            n172 = local write "fitCol"(w201) -> ()
          }
        }
        n173 = case shown="True" w140 {
          tunnel: w147 -> [_ w200]
          frame False {
          }
          frame True {
            n174 = local write "fitRow"(w200) -> ()
          }
        }
      }
      event "device": Value Change {
        n175 = event-data() -> ()  [unwired: 1 in, 6 out]
        n176 = flat-sequence {
          tunnel: [w247] -> w229
          tunnel: w229 -> [w251]
          tunnel: [w251] -> w228
          tunnel: w228 -> [w266]
          tunnel: [w266] -> w230
          tunnel: w230 -> [w270]
          frame #0 {
            w236 = dbl[][] [[0.0, 0.0, 0.0, 0.0], [0.0, 0.0, 0.0, 0.0], [0.0, 0.0, 0.0, 0.0], [0.0, 0.0, 0.0, 0.0]] ("horizontalFitCovariance")
            w237 = dbl[] [0.0, 0.0, 0.0, 0.0, 0.0] ("horizontalBestFitPars")
            w234 = FALSE
            n177 = local read "nbits"() -> (w231:u16)
            n178 = local write "horizontalFitCovariance"(w236) -> ()
            n179 = local write "horizontalBestFitPars"(w237) -> ()
            n180 = local write "verticalFitCovariance"(w236) -> ()
            n181 = local write "exposureTimeStatus"(w234) -> ()
            n182 = Logical Shift(y=w231, x=i16 1 ("y")) -> (x << y=w232:i16)
            n183 = local write "horizontalFitButton"(w234) -> ()
            n184 = local write "saveCurrentImage"(w234) -> ()
            n185 = local write "verticalBestFitPars"(w237) -> ()
            n186 = local write "maxTrialNumber"(5 ("maxTrialNumber")) -> ()
            n187 = local write "verticalFitButton"(w234) -> ()
            n188 = local write "last log filename"("" ("last Image filename")) -> ()
            n189 = local write "runChartButton"(w234) -> ()
            n190 = local write "TDMS_Location"(path "" ("TDMS_Location")) -> ()
            n191 = local write "logDataButton"(w234) -> ()
            n192 = local write "intensityRangeMax"(w232) -> ()
            n193 = local write "followCx"(w234) -> ()
            n194 = local write "followCy"(w234) -> ()
          }
          frame #1 {
            n195 = local read "cameraSession"() -> (w241:T4)
            n196 = call <vilib>:"IMAQdx Close Camera.vi"("Session In"=w241) -> ("error out"=w240:errorcluster)  [unwired: 10 in]
            n197 = local write "errorCameraConfig"(w240) -> ()
          }
          frame #2 {
            n198 = local read "device"() -> (w242:string)
            n199 = call <vilib>:"IMAQdx Open Camera.vi"("Session In"=w242) -> ("error out"=w250:errorcluster, "Session Out"=w248:T4)  [unwired: 9 in]
            n200 = Format Into String(format string="Accessing and configuring  camera \"%s\" ..." ("string"), w242) -> (resulting string=w245:string)  [unwired: 2 in, 1 out]
            n201 = call "temporaryMessage.vi"("milliseconds to wait"=u32 1000, "message"=w245) -> ()  [unwired: 1 in]
            n202 = call <vilib>:"IMAQdx Configure Grab.vi"("error in"=w250, "Number of Buffers"=u32 2, "Session In"=w248) -> ("error out"=w246:errorcluster, "Session Out"=w247:T4)  [unwired: 7 in]
            n203 = local write "errorCameraConfig"(w246) -> ()
          }
          frame #3 {
            n204 = call "getCameraParameters.vi"("IMAQdx Session"=w251) -> ("errorCameraParsRequest"=w252:errorcluster, "VendorNameModelName"=w254:string, "IPAddress"=w253:string)  [unwired: 8 in]
            n205 = local write "vendorNameModelName"(w254) -> ()
            n206 = local write "errorCameraParsRequest"(w252) -> ()
            n207 = local write "IPAddress"(w253) -> ()
          }
          frame #4 {
            n208 = local read "imageViewer"() -> (w265:T2)
            n209 = call "imageParameters.vi"("sessionIn"=w266, "imageIn"=w265) -> ("imageHalfRows"=w255:i32, "imageHalfCols"=w256:i32, "imageCols"=w257:i32, "imageRows"=w258:i32, "errorImageGrab"=w267:errorcluster)  [unwired: 5 in]
            n210 = local write "errorImageGrab"(w267) -> ()
            n211 = local write "imageRows"(w258) -> ()
            n212 = local write "rowsOffset"(w255) -> ()
            n213 = local write "imageCols"(w257) -> ()
            n214 = local write "colsOffset"(w256) -> ()
            n215 = local write "fitRow"(w255) -> ()
            n216 = local write "fitCol"(w256) -> ()
            n217 = local read "plotUnitsPrefix"() -> (w259:dbl)
            n218 = local read "pixelSize"() -> (w260:dbl)
            n219 = call "axisParameters.vi"("colOffset"=w256, "rowOffset"=w255, "cols"=w257, "rows"=w258, "pixelSize"=w260, "plotUnitsPrefix"=w259) -> ("yAxisScaled"=w261:dbl[], "xAxisScaled"=w263:dbl[], "yAxis"=w262:dbl[], "xAxis"=w264:dbl[])
            n220 = local write "xAxis"(w264) -> ()
            n221 = local write "xAxisScaled"(w263) -> ()
            n222 = local write "yAxis"(w262) -> ()
            n223 = local write "yAxisScaled"(w261) -> ()
          }
          frame #5 {
            n224 = local read "exposuretimeUnitsPrefix"() -> (w269:dbl)
            n225 = call "exposureTimeGet.vi"("exposureUnitsPrefix"=w269, "Session in"=w270) -> ("errorOut"=w268:errorcluster, "exposureTime"=w271:dbl)  [unwired: 2 in]
            n226 = local write "exposureTime"(w271) -> ()
            n227 = local write "errorExposureTime"(w268) -> ()
          }
        }
      }
      event "setOrigin": Value Change {
        n228 = event-data() -> ()  [unwired: 1 in, 6 out]
        n229 = local read "imageCols"() -> (w272:i32)
        n230 = local read "fitCol"() -> (w274:i32)
        n231 = local read "plotUnitsPrefix"() -> (w276:dbl)
        n232 = local read "fitRow"() -> (w275:i32)
        n233 = local read "pixelSize"() -> (w277:dbl)
        n234 = local read "imageRows"() -> (w273:i32)
        n235 = local write "colsOffset"(w274) -> ()
        n236 = local write "rowsOffset"(w275) -> ()
        n237 = call "axisParameters.vi"("colOffset"=w274, "rowOffset"=w275, "cols"=w272, "rows"=w273, "pixelSize"=w277, "plotUnitsPrefix"=w276) -> ("yAxisScaled"=w279:dbl[], "xAxisScaled"=w281:dbl[], "yAxis"=w280:dbl[], "xAxis"=w278:dbl[])
        n238 = local write "xAxisScaled"(w281) -> ()
        n239 = local write "yAxisScaled"(w279) -> ()
        n240 = local write "xAxis"(w278) -> ()
        n241 = local write "yAxis"(w280) -> ()
      }
      event "resetOrigin": Value Change {
        n242 = event-data() -> ()  [unwired: 1 in, 6 out]
        n243 = local read "plotUnitsPrefix"() -> (w288:dbl)
        n244 = local read "imageRows"() -> (w286:i32)
        n245 = local read "imageCols"() -> (w282:i32)
        n246 = local read "pixelSize"() -> (w289:dbl)
        n247 = Logical Shift(y=i16 -1, x=w286) -> (x << y=w287:i32)
        n248 = Logical Shift(y=i16 -1, x=w282) -> (x << y=w283:i32)
        n249 = call "axisParameters.vi"("colOffset"=w283, "rowOffset"=w287, "cols"=w282, "rows"=w286, "pixelSize"=w289, "plotUnitsPrefix"=w288) -> ("yAxisScaled"=w290:dbl[], "xAxisScaled"=w292:dbl[], "yAxis"=w291:dbl[], "xAxis"=w293:dbl[])
        n250 = local write "xAxisScaled"(w292) -> ()
        n251 = local write "yAxisScaled"(w290) -> ()
        n252 = local write "xAxis"(w293) -> ()
        n253 = local write "yAxis"(w291) -> ()
      }
      event "nbits": Value Change {
        n254 = event-data() -> ()  [unwired: 1 in, 6 out]
        n255 = local read "nbits"() -> (w296:u16)
        n256 = Logical Shift(y=w296, x=i16 1 ("y")) -> (x << y=w294:i16)
        n257 = local write "intensityRangeMax"(w294) -> ()
      }
      event "units", "pixelSize": Value Change {
        n258 = event-data() -> ()  [unwired: 1 in, 6 out]
        n259 = case shown="\"um\"" "units" {
          tunnel: [1000000.0 1000.0 100.0] -> w305
          tunnel: ["um" "mm" "cm"] -> w307
          frame "um" {
          }
          frame "mm" {
          }
          frame "cm" {
          }
        }
        n260 = local read "colsOffset"() -> (w297:i32)
        n261 = local read "rowsOffset"() -> (w298:i32)
        n262 = local read "imageRows"() -> (w304:i32)
        n263 = local read "imageCols"() -> (w303:i32)
        n264 = local write "plotUnitsPrefix"(w305) -> ()
        n265 = local read "pixelSize"() -> (w306:dbl)
        n266 = call "axisParameters.vi"("colOffset"=w297, "rowOffset"=w298, "cols"=w303, "rows"=w304, "pixelSize"=w306, "plotUnitsPrefix"=w305) -> ("yAxisScaled"=w299:dbl[], "xAxisScaled"=w301:dbl[], "yAxis"=w300:dbl[], "xAxis"=w302:dbl[])
        n267 = Format Into String(format string="Horizontal Coordinate, x [%s]", w307) -> (resulting string=w314:string)  [unwired: 2 in, 1 out]
        n268 = Format Into String(format string="Vertical  Coordinate, x [%s]", w307) -> (resulting string=w315:string)  [unwired: 2 in, 1 out]
        n269 = Format Into String(format string="Centroid Horizontal Coordinate, Cx   [%s]", w307) -> (resulting string=w308:string)  [unwired: 2 in, 1 out]
        n270 = Format Into String(format string="Spot radii , wx wy , [%s]", w307) -> (resulting string=w309:string)  [unwired: 2 in, 1 out]
        n271 = Format Into String(format string="Centroid Vertical Coordinate, Cy   [%s]", w307) -> (resulting string=w310:string)  [unwired: 2 in, 1 out]
        n272 = property on="CyPlot" class="WFChart (strict)"("YScale.NameLbl.Text"=w310) -> ()  [unwired: 2 in, 2 out]
        n273 = property on="horizontal FitPlot" class="XYGraph (strict)"("XScale.NameLbl.Text"=w314) -> ()  [unwired: 2 in, 2 out]
        n274 = property on="CxPlot" class="WFChart (strict)"("YScale.NameLbl.Text"=w308) -> ()  [unwired: 2 in, 2 out]
        n275 = local write "xAxisScaled"(w301) -> ()
        n276 = local write "yAxisScaled"(w299) -> ()
        n277 = property on="verticalFitPlot" class="XYGraph (strict)"("YScale.NameLbl.Text"=w315) -> ()  [unwired: 2 in, 2 out]
        n278 = property on="wx_wyPlot" class="WFChart (strict)"("YScale.NameLbl.Text"=w309) -> ()  [unwired: 2 in, 2 out]
        n279 = local write "xAxis"(w302) -> ()
        n280 = local write "yAxis"(w300) -> ()
      }
      event "aboutButton": Value Change {
        n281 = event-data() -> ()  [unwired: 1 in, 1 out]
        n282 = call "About Message"() -> ()  [unwired: 10 in, 2 out]
      }
      event "logDataButton": Value Change {
        n283 = event-data() -> ()  [unwired: 1 in, 1 out]
        n284 = local read "logDataButton"() -> (w325:bool)
        n285 = feedback #2() -> (w326:refnum<k34>)  [unwired: 1 in]
        n286 = case shown="True" w325 {
          tunnel: [w331 w332] -> w327
          tunnel: w326 -> [w331 _]
          frame False {
            n287 = TDMS Close(11:w331) -> (0:w329:errorcluster, 3:w330:path)  [unwired: 1 in]
            n288 = call <vilib>:"TDMS - File Viewer (NXG Style).vi"("error in"=w329, "file in"=w330) -> ("error out"=→"errorTDMS_LogClose":errorcluster)  [unwired: 8 in, 1 out]
          }
          frame True {
            n289 = flat-sequence {
              tunnel: [w337] -> w333
              tunnel: w333 -> [w341]
              tunnel: [w343] -> w332
              frame #0 {
                n290 = call "TDMS_Location.vi"("baseName"="logBaseName", "basePath"="log basePath") -> ("location"=w337:path, "filenname"=→"last log filename":string)  [unwired: 2 in]
                "TDMS_Location" <- w337
                n291 = local write "horizontalFitButton"(TRUE ("horizontalFitButton")) -> ()
                n292 = local write "verticalFitButton"(TRUE ("verticalFitButton")) -> ()
              }
              frame #1 {
                n293 = TDMS Open(6:FALSE ("disable buffering? (T)"), 10:T7."create" ("operation (0:open)"), 11:w341) -> (0:w342:errorcluster, 3:w343:refnum<k34>)  [unwired: 4 in]
                "errorTDMS_LogOpen" <- w342
                "TDMS_Handle" <- w343
                n294 = call "TDMS_FileLocationErrorMessage.vi"("fileLocation"=w341, "errorIn"=w342) -> ("buttonStatus"=w340:bool)  [unwired: 8 in, 1 out]
                n295 = local write "logDataButton"(w340) -> ()
              }
            }
          }
        }
        n296 = feedback-in #2(w327) -> ()
      }
      event "runChartButton": Value Change {
        w346 = TRUE ("horizontalFitButton")
        n297 = event-data() -> ()  [unwired: 1 in, 6 out]
        n298 = local write "horizontalFitButton"(w346) -> ()
        n299 = local write "verticalFitButton"(w346) -> ()
      }
      event "saveCurrentImage", "baseName": Value Change {
        n300 = event-data() -> ()  [unwired: 1 in, 1 out]
        n301 = flat-sequence {
          tunnel: [w357] -> w349
          tunnel: [w352] -> w347
          tunnel: [w363] -> w351
          tunnel: [w362] -> w350
          tunnel: w349 -> [w368]
          tunnel: [w368] -> w348
          tunnel: w347 -> [w364]
          tunnel: w351 -> [w371]
          tunnel: w350 -> [w370]
          tunnel: w348 -> [w369]
          frame #0 {
            n302 = local read "exposureTime"() -> (w354:dbl)
            n303 = local write "saveCurrentImage"(FALSE ("saveCurrentImage")) -> ()
            n304 = call "imageLocation.vi"("extension"="png", "exposureTime"=w354, "baseName"="baseName", "basePath"="basePath") -> ("imageLocation"=w352:path, "imageLocationString"=w357:string)
            "last Image filename" <- w357
            n305 = Format Into String(format string="saving image \"%s\" ..." ("string"), w357) -> (resulting string=w355:string)  [unwired: 2 in, 1 out]
            n306 = call "temporaryMessage.vi"("milliseconds to wait"=u32 400, "message"=w355) -> ()  [unwired: 1 in]
          }
          frame #1 {
            n307 = local read "imageViewer"() -> (w366:T2)
            n308 = call-poly "IMAQ Write File 2"("Use bit depth? (false)"=TRUE, "File Path"=w364, "Image"=w366) -> ("error out"=w367:errorcluster)  [unwired: 7 in, 1 out]
            n309 = Unbundle By Name(w367) -> ("status"=w363:bool, "code"=w362:i32)
          }
          frame #2 {
            n310 = case shown="True" w371 {
              tunnel: w369 -> [_ w373]
              tunnel: w370 -> [_ w372]
              frame False {
              }
              frame True {
                n311 = Format Into String(format string="Error: cannot save image \"%s\", error code  %ld .", w373, w372) -> (resulting string=w374:string)  [unwired: 2 in, 1 out]
                n312 = One Button Dialog(message=w374) -> ()  [unwired: 1 in, 1 out]
              }
            }
          }
        }
      }
      event "stop": Value Change {
        n313 = event-data() -> ()  [unwired: 1 in, 1 out]
      }
    }
  }
  n314 = call <vilib>:"IMAQdx Close Camera.vi"("Session In"=w1) -> ()  [unwired: 10 in, 1 out]
